vi "Set Wheel Parameters.vi"(8 "error in (no error)":errorcluster, 9 "wheel name":string, 10 "wheel parameters":T1={"wheel radius"=1.0, "gear ratio"=1.0, "forward rotation direction"=0} {"forward rotation direction" items=["Clockwise", "Counterclockwise"]}, 11 "wheel in":refnum<class "NI_Robotics_Wheel.lvclass">) -> (0 "error out":errorcluster, 3 "wheel out":refnum<class "NI_Robotics_Wheel.lvclass">)   [LabVIEW 2017, in "NI_Robotics_Wheel.lvclass"]
uses:
  <vilib>/robotics/Steering/Wheel/NI_Robotics_Wheel.lvclass
  <vilib>/robotics/Steering/Wheel/Wheel Parameters.ctl
  <vilib>/robotics/Steering/Wheel/Rotation Direction.ctl
  <vilib>/robotics/Steering/Wheel/NI_Robotics_Wheel.lvclass/NI_Robotics_Wheel.ctl
  <vilib>/robotics/Utilities/Generate Error.vi
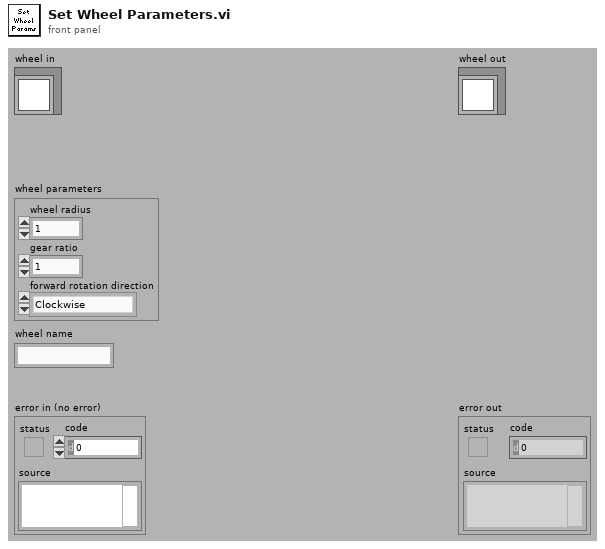
[diagram p1: front panel]
types:
  T1 = typedef "NI_Robotics_Wheel.lvclass/Wheel Parameters.ctl" = cluster{"wheel radius":dbl, "gear ratio":dbl, "forward rotation direction":T2}
  T2 = typedef "NI_Robotics_Wheel.lvclass/Rotation Direction.ctl" = u16
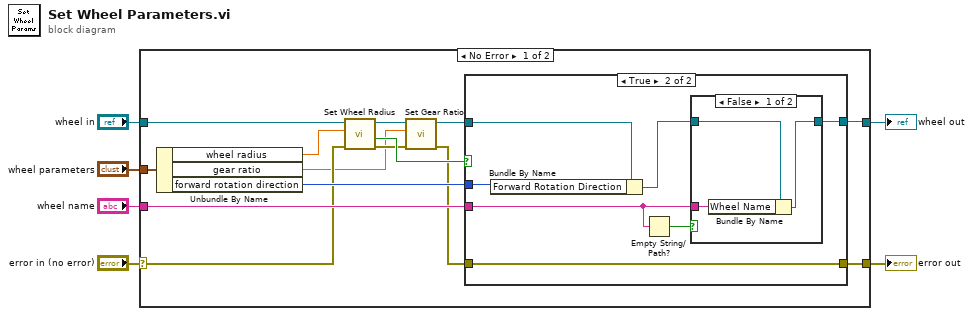
[diagram p0: block diagram]
diagram:
  n1 = case shown="No Error" "error in (no error)" {
    selector: "error in (no error)" -> [w13 w35]
    tunnel: [w16 w35] -> w5
    tunnel: [w17 w34] -> w3
    tunnel: "wheel in" -> [w15 w34]
    tunnel: "wheel parameters" -> [w20 _]
    tunnel: "wheel name" -> [w18 _]
    frame No Error {
      n2 = Unbundle By Name(w20) -> ("wheel radius"=w14:dbl, "gear ratio"=w7:dbl, "forward rotation direction"=w19:T2)
      n3 = call <vilib>:"Set Wheel Radius.vi"("error in (no error)"=w13, "wheel radius"=w14, "wheel in"=w15) -> ("error out"=w9:errorcluster, "valid?"=w12:bool, "wheel out"=w11:refnum<class "NI_Robotics_Wheel.lvclass">)  [unwired: 6 in]
      n4 = call <vilib>:"Set Gear Ratio.vi"("error in (no error)"=w9, "gear ratio"=w7, "wheel in"=w11) -> ("error out"=w8:errorcluster, "wheel out"=w10:refnum<class "NI_Robotics_Wheel.lvclass">)  [unwired: 7 in]
      n5 = case shown="True" w12 {
        tunnel: w19 -> [_ w29]
        tunnel: w10 -> [w22 w28]
        tunnel: w18 -> [_ w26]
        tunnel: [w22 w24] -> w17
        tunnel: w8 -> [w21 w23]
        tunnel: [w21 w23] -> w16
        frame False {
        }
        frame True {
          n6 = Bundle By Name(cluster=w28, "Forward Rotation Direction"=w29) -> (w25:refnum<class "NI_Robotics_Wheel.lvclass">)
          n7 = Empty String/Path?(string/path=w26) -> (empty?=w27:bool)
          n8 = case shown="False" w27 {
            tunnel: w26 -> [w31 _]
            tunnel: w25 -> [w32 w33]
            tunnel: [w30 w33] -> w24
            frame False {
              n9 = Bundle By Name(cluster=w32, "Wheel Name"=w31) -> (w30:refnum<class "NI_Robotics_Wheel.lvclass">)
            }
            frame True {
            }
          }
        }
      }
    }
    frame Error {
    }
  }
  "error out" <- w5
  "wheel out" <- w3
